vi "圆十字标注.vi"(9 "Color":u32(colorbox)=16711680, 10 "簇":cluster{"X":dbl, "Y":dbl}, 11 "引用句柄输入":T1) -> (3 "引用句柄输出":T1)   [LabVIEW 2014]
uses:
  <vilib>/vision/Image Controls.llb/IMAQ Image.ctl
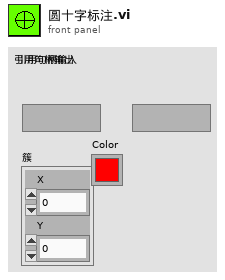
[diagram p1: front panel]
types:
  T1 = typedef "IMAQ Image.ctl" = refnum<image>
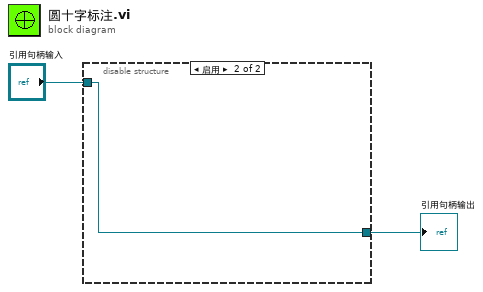
[diagram p0: block diagram]
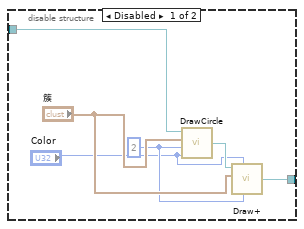
[diagram p2: hidden frame]
diagram:
  n1 = disable-structure shown="启用" {
    disable-tunnel: [w7 w9] -> w2
    disable-tunnel: "引用句柄输入" -> [w4 w9]
    frame Disabled {
      w5 = 2 ("Circle_D")
      n2 = call "DrawCircle.vi"("Color"="Color", "Circle_D"=w5, "CircleCenterPosition"="簇", "Img in"=w4) -> ("Img out"=w6:T1)
      n3 = call "Draw+.vi"("Width"=w5, "Color"="Color", "input cluster"="簇", "Image In"=w6) -> ("Image Out"=w7:T1)  [unwired: 2 in]
    }
    frame Enabled {
    }
  }
  "引用句柄输出" <- w2
